vi "Database.Changeover.vi"(7 "Idx":i32, 8 "error in":errorcluster, 10 "Ref":string, 11 "Data in":T1) -> (0 "error out":errorcluster, 3 "Data out":T1)   [LabVIEW 2016]
doc: "Connect to database\n\nWabco 2017 All right reserved\nAuthor: maciej.szupienko@wabco-auto.com"
uses:
  Database.Data.ctl
  Database.Data.Status.ctl
  Database.Data.Sets.ctl
  Cache/Cache.TestSteps.Fglb.Action.ctl
  Cache/Cache.TestSteps.Fglb.TestData.ctl
  ProdaNG/Controls/ProdaNG.Process.ctl
  ProdaNG/Controls/ProdaNG.ProcessStep.ctl
  ProdaNG/Controls/ProdaNG.ProcessStepParam.ctl
  ProdaNG/Controls/ProdaNG.TestStep.ctl
  ProdaNG/Controls/ProdaNG.TestValue.ctl
  ProdaNG/Controls/ProdaNG.TestStepParam.ctl
  ProdaNG/Controls/ProdaNG.Unit.ctl
  Cache/Cache.TestSteps.Fglb.ResultData.ctl
  ProdaNG/Controls/ProdaNG.ProcessResult.ctl
  ProdaNG/Controls/ProdaNG.ProcessStepResult.ctl
  ProdaNG/Controls/ProdaNG.TestStepResult.ctl
  ProdaNG/Controls/ProdaNG.TestValueResult.ctl
  Tools/Translator/Translator.Message.ctl
  Tools/EventLog/EventLog.EventSource.ctl
  Tools/EventLog/EventLog.New(single).vi
  Global/ApplicationGlobal.vi
  Tools/EventLog/EventLog.Buffer.vi
  Tools/EventLog/EventLog.File.ReadWrite.vi
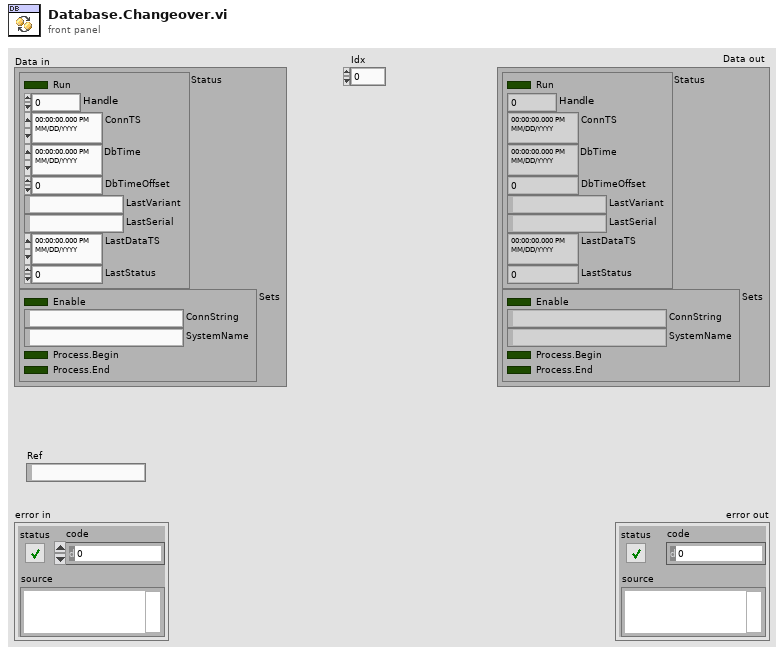
[diagram p1: front panel]
types:
  T1 = typedef "Database.Data.ctl" = cluster{"Status":T2, "Sets":T3}
  T2 = typedef "Database.Data.Status.ctl" = cluster{"Run":bool, "Handle":i32, "ConnTS":timestamp, "DbTime":timestamp, "DbTimeOffset":dbl, "LastVariant":string, "LastSerial":string, "LastDataTS":timestamp, "LastStatus":i32}
  T3 = typedef "Database.Data.Sets.ctl" = cluster{"Enable":bool, "ConnString":string, "SystemName":string, "Process.Begin":bool, "Process.End":bool}
  T4 = typedef "EventLog.EventSource.ctl" = enum16{"All", "Gui", "Cache", "PLC1", "PLC2", "PLC3", "DB", "DB01", "DB02", "DB03", "DB04", "DB05", "DB06", "DB07", "DB08", "DB09", "DB10", "DB11", "DB12", "DB13", "DB14", "DB15", "DB16"}
  T5 = typedef "Translator.Message.ctl" = enum16{"-", "Event confirmed", "Log out", "Log in", "Shutdown", "Cancel", "Start", "Continue", "Stop", "On", "Off", "OK", "NOK", "NOK %s", "This", "Prev", "Home", "Work", "In progress...", "Missing", "Empty", "Hardware failure", "Initial", "Error %d >> %s", "Error %d >> %s >> %s", "Starting %s", "Quitting %s", "Configured", "Initializing", "Quitting", "Loading", "Running %s", "Stopped", "Summary", "Do you want to continue?", "Do you want to exit?", "Log out?", "System", "All", "IDLE", "Translating...%s", "Not found", "Alarm %s", "Run", "Skip", "Abort", "Repeat", "Please wait...", "Database disconnected", "Login to database successful", "Login to database failed: %d; %s", "Get process step data for %s", "Changeover off", "Changeover into %s", "Product %s | %s found in cache with status %d at previous station", "Product %s | %s found in database with status %d at previous station", "Product %s | %s not found in cache at previous station", "Product %s | %s not found in database at previous station", "Product %s | %s found in cache with status %d at this station (%d repetion)", "Product %s | %s found in database with status %d at this station (%d repetition)", "Product %s | %s not found in cache at this station", "Product %s | %s not found in database at this station", "Product %s | %s found in cache for component %s | %s", "Product %s | %s found in database for component %s | %s", "Product not found in cache for component %s | %s", "Product not found in database for component %s | %s", "Product %s | %s connected with component %s | %s (cache)", "Product %s | %s connected with component %s | %s (database)", "New data for %s | %s (cache)", "New data for %s | %s (database)", "File %s moved (cache)", "File %s deleted (cache)", "Msg %d >> %s", "PLC LifeBit Failure", "Reconnecting DB", "Reconnecting PLC", "Free disk space is below 1GB - contact technician"}
  T6 = typedef "Cache.TestSteps.Fglb.ResultData.ctl" = cluster{"File":path, "Ref":string, "Serial":string, "Pr":T7, "PSr":T8, "TSr":cluster{"TSr":T9, "TVr":T10[]}[]}
  T7 = typedef "ProdaNG.ProcessResult.ctl" = cluster{"c_id":string, "productId":string, "processId":i32, "statusId":i32, "startTime":string, "endTime":string}
  T8 = typedef "ProdaNG.ProcessStepResult.ctl" = cluster{"c_id":string, "processResultId":string, "processStepId":i32, "statusId":i32, "operatorId":i32, "startTime":string, "endTime":string}
  T9 = typedef "ProdaNG.TestStepResult.ctl" = cluster{"c_id":string, "processStepResultId":string, "testStepId":i32, "statusId":i32}
  T10 = typedef "ProdaNG.TestValueResult.ctl" = cluster{"c_id":string, "testStepResultId":string, "testValueId":i32, "result":dbl, "statusId":i32, "contentId":string}
  T11 = typedef "Cache.TestSteps.Fglb.TestData.ctl" = cluster{"Ref":string, "Desc":string, "P":T12, "PS":T13, "PP":T14[], "TS":cluster{"TS":T15, "TV":T16[], "TP":T17[]}[], "Units":T18[]}
  T12 = typedef "ProdaNG.Process.ctl" = cluster{"i_id":i32, "productionLineId":i32, "releaseId":i32, "contentId":string, "previewId":string, "mdReason":string, "mdUser":string, "mdTime":string, "description":string}
  T13 = typedef "ProdaNG.ProcessStep.ctl" = cluster{"i_id":i32, "processId":i32, "systemId":i32, "releaseId":i32, "processSequence":i32, "limitYellow":dbl, "limitRed":dbl, "mdReason":string, "mdUser":string, "mdTime":string, "filename":string, "transfer":string, "description":string}
  T14 = typedef "ProdaNG.ProcessStepParam.ctl" = cluster{"i_id":i32, "processStepId":i32, "unitId":i32, "contentId":string, "previewId":string, "value":dbl, "valueText":string, "paramSequence":i32, "history":i32, "mdReason":string, "mdUser":string, "mdTime":string, "description":string}
  T15 = typedef "ProdaNG.TestStep.ctl" = cluster{"i_id":i32, "processStepId":i32, "testSequence":i32, "testOrder":i32, "mdReason":string, "mdUser":string, "mdTime":string, "description":string}
  T16 = typedef "ProdaNG.TestValue.ctl" = cluster{"i_id":i32, "testStepId":i32, "releaseId":i32, "unitId":i32, "contentId":string, "previewId":string, "maximum":dbl, "minimum":dbl, "valueText":string, "testValueSequence":i32, "history":i32, "mdReason":string, "mdUser":string, "mdTime":string, "description":string}
  T17 = typedef "ProdaNG.TestStepParam.ctl" = cluster{"i_id":i32, "testStepId":i32, "unitId":i32, "contentId":string, "previewId":string, "value":dbl, "valueText":string, "paramSequence":i32, "history":i32, "mdReason":string, "mdUser":string, "mdTime":string, "description":string}
  T18 = typedef "ProdaNG.Unit.ctl" = cluster{"i_id":i32, "name":string, "mdReason":string, "mdUser":string, "mdTime":string, "description":string}
  T19 = typedef "Cache.TestSteps.Fglb.Action.ctl" = enum16{"init", "add", "get"}
  T20 = typedef "Database.Data.Variant.Sets.ctl" = cluster{"PrevStations":string[], "ThisStations":string[]}
  T21 = typedef "ProdaNG.Identification.ctl" = cluster{"processId":i32, "systemId":i32, "processStepId":i32, "wabcoPartId":i32}
  T22 = cluster{"TestStep":T15, "TestStepValues":T16[], "TestStepParams":T17[]}
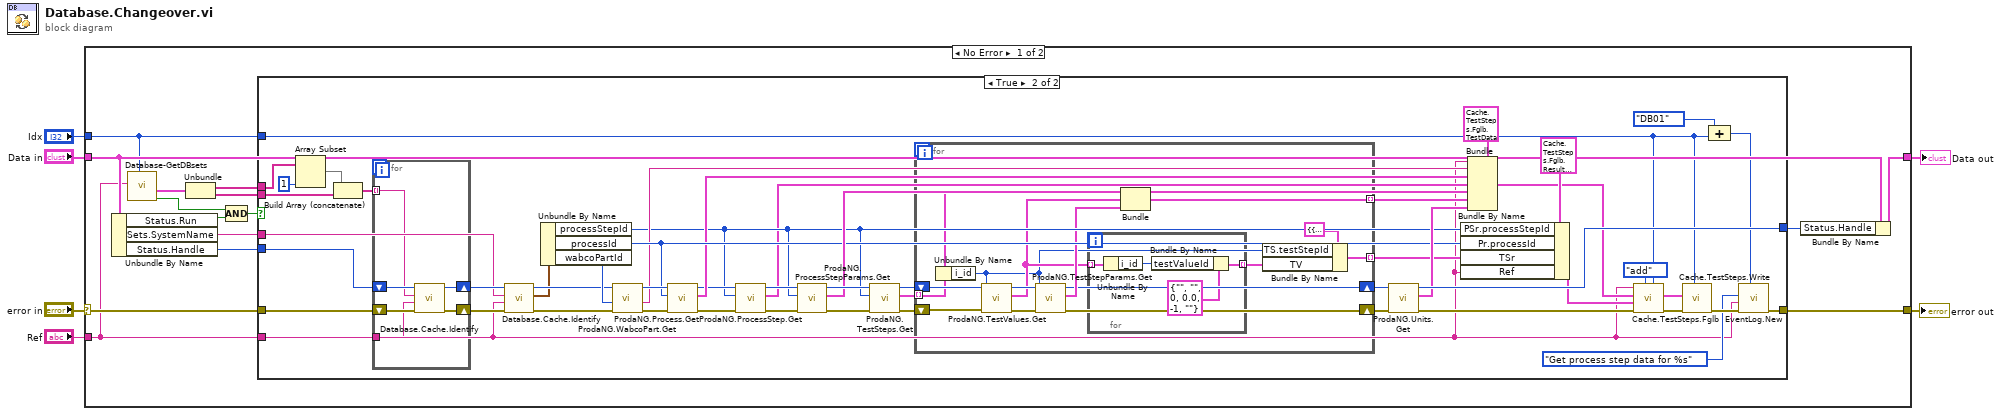
[diagram p0: block diagram]
diagram:
  n1 = case shown="No Error" "error in" {
    selector: "error in" -> [w21 w101]
    tunnel: [w7 w101] -> w6
    tunnel: "Data in" -> [w18 w100]
    tunnel: "Idx" -> [w8 _]
    tunnel: [w16 w100] -> w2
    tunnel: "Ref" -> [w12 _]
    frame No Error {
      n2 = Unbundle By Name(w18) -> ("Status.Run"=w11:bool, "Sets.SystemName"=w20:string, "Status.Handle"=w19:i32)
      n3 = call "Database-GetDBsets.vi"("Idx"=w8, "Variant"=w12) -> ("Found"=w10:bool, "Variant Sets"=w15:T20)  [unwired: 5 in, 3 out]
      n4 = Unbundle(w15) -> ("PrevStations"=w14:string[], "ThisStations"=w13:string[])
      n5 = Compound Arithmetic op=AND(w10, w11) -> (w9:bool)
      n6 = case shown="True" w9 {
        tunnel: w21 -> [w22 w43]
        tunnel: [w22 w29] -> w7
        tunnel: w14 -> [_ w33]
        tunnel: w20 -> [_ w34]
        tunnel: w19 -> [w23 w40]
        tunnel: [w23 w75] -> w17
        tunnel: w13 -> [_ w42]
        tunnel: w12 -> [_ w24]
        tunnel: w8 -> [_ w27]
        frame False {
        }
        frame True {
          n7 = Array Subset(array=w33, length=1) -> (w32:string[])  [unwired: 1 in]
          n8 = Build Array (concatenate)(w32, w42) -> (w41:string[])
          n9 = for {
            tunnel: w41 -> [w76] mode=indexing
            shift-right: [w80] -> w38
            shift-left: w40 -> [w79]
            tunnel: w24 -> [w77]
            shift-right: [w81] -> w39
            shift-left: w43 -> [w78]
            n10 = call "Database.Cache.Identify.vi"("error in (no error)"=w78, "Variant"=w77, "SystemName"=w76, "DB Handle in"=w79) -> ("error out"=w81:errorcluster, "DB Handle out"=w80:i32)  [unwired: 5 in, 1 out]
          }
          n11 = call "Database.Cache.Identify.vi"("error in (no error)"=w39, "Variant"=w24, "SystemName"=w34, "DB Handle in"=w38) -> ("error out"=w37:errorcluster, "SytemID"=w35:T21, "DB Handle out"=w36:i32)  [unwired: 5 in]
          n12 = Unbundle By Name(w35) -> ("processStepId"=w45:i32, "processId"=w55:i32, "wabcoPartId"=w74:i32)
          n13 = call "ProdaNG.WabcoPart.Get.vi"("error in (no error)"=w37, "WabcoPartId (-1: use WabcoNumber)"=w74, "dbHandleIn"=w36) -> ("error out"=w72:errorcluster, "ProductName"=w52:string, "dbHandle"=w73:i32)  [unwired: 5 in, 1 out]
          n14 = call "ProdaNG.Process.Get.vi"("error in (no error)"=w72, "processId"=w55, "dbHandleIn"=w73) -> ("error out"=w48:errorcluster, "Process"=w53:T12, "dbHandle"=w49:i32)  [unwired: 5 in, 1 out]
          n15 = call "ProdaNG.ProcessStep.Get.vi"("error in (no error)"=w48, "processStepId"=w45, "dbHandleIn"=w49) -> ("error out"=w47:errorcluster, "ProcessStep"=w44:T13, "dbHandle"=w46:i32)  [unwired: 6 in]
          n16 = call "ProdaNG.ProcessStepParams.Get.vi"("error in (no error)"=w47, "processStepId"=w45, "dbHandleIn"=w46) -> ("error out"=w70:errorcluster, "ProcStepParams"=w60:T14[], "dbHandle"=w69:i32)  [unwired: 6 in]
          n17 = call "ProdaNG.TestSteps.Get.vi"("error in (no error)"=w70, "processStepId"=w45, "dbHandleIn"=w69) -> ("error out"=w68:errorcluster, "TestSteps"=w66:T15[], "dbHandle"=w67:i32)  [unwired: 6 in]
          n18 = for {
            shift-right: [w91] -> w64
            shift-left: w68 -> [w95]
            tunnel: w66 -> [w83] mode=indexing
            tunnel: [w90] -> w65 mode=indexing
            tunnel: [w84] -> w56 mode=indexing
            shift-right: [w82] -> w63
            shift-left: w67 -> [w94]
            n19 = Unbundle By Name(w83) -> ("i_id"=w86:i32)
            n20 = call "ProdaNG.TestValues.Get.vi"("error in (no error)"=w95, "testStepId"=w86, "dbHandleIn"=w94) -> ("error out"=w92:errorcluster, "TestStepValues"=w87:T16[], "dbHandle"=w93:i32)  [unwired: 6 in]
            n21 = call "ProdaNG.TestStepParams.Get.vi"("error in (no error)"=w92, "testStepId"=w86, "dbHandleIn"=w93) -> ("error out"=w91:errorcluster, "TestStepParams"=w89:T17[], "dbHandle"=w82:i32)  [unwired: 6 in]
            n22 = for {
              tunnel: w87 -> [w99] mode=indexing
              tunnel: [w96] -> w88 mode=indexing
              n23 = Unbundle By Name(w99) -> ("i_id"=w98:i32)
              n24 = Bundle By Name(cluster=T10 {"c_id"="", "testStepResultId"="", "testValueId"=0, "result"=0.0, "statusId"=-1, "contentId"=""} ("TV"), "testValueId"=w98) -> (w96:T10)
            }
            n25 = Bundle("TestStep"=w83, "TestStepValues"=w87, "TestStepParams"=w89) -> (w90:T22)  [unwired: 1 in]
            n26 = Bundle By Name(cluster=cluster{"TS":T9, "TV":T10[]} {"TS"={"c_id"="", "processStepResultId"="", "testStepId"=0, "statusId"=-1}, "TV"=[]} ("Cluster"), "TS.testStepId"=w86, "TV"=w88) -> (w84:cluster{"TS":T9, "TV":T10[]})
          }
          n27 = call "ProdaNG.Units.Get.vi"("error in (no error)"=w64, "dbHandleIn"=w63) -> ("error out"=w57:errorcluster, "units"=w62:T18[], "dbHandle"=w75:i32)  [unwired: 6 in, 1 out]
          n28 = Bundle By Name(cluster=T6 {"File"=path "", "Ref"="", "Serial"="", "Pr"={"c_id"="", "productId"="", "processId"=0, "statusId"=0, "startTime"="", "endTime"=""}, "PSr"={"c_id"="", "processResultId"="", "processStepId"=0, "statusId"=0, "operatorId"=0, "startTime"="", "endTime"=""}, "TSr"=[]} ("Result in"), "PSr.processStepId"=w45, "Pr.processId"=w55, "TSr"=w56, "Ref"=w24) -> (w58:T6)
          n29 = Bundle(cluster=T11 {"Ref"="", "Desc"="", "P"={"i_id"=0, "productionLineId"=0, "releaseId"=0, "contentId"="", "previewId"="", "mdReason"="", "mdUser"="", "mdTime"="", "description"=""}, "PS"={"i_id"=0, "processId"=0, "systemId"=0, "releaseId"=0, "processSequence"=0, "limitYellow"=0.0, "limitRed"=0.0, "mdReason"="", "mdUser"="", "mdTime"="", "filename"="", "transfer"="", "description"=""}, "PP"=[], "TS"=[], "Units"=[]} ("TestStep in"), "Ref"=w24, "Desc"=w52, "P"=w53, "PS"=w44, "PP"=w60, "TS"=w65, "Units"=w62) -> (w54:T11)
          n30 = call "Cache.TestSteps.Fglb.vi"("SystemIdx"=w27, "Action (get)"=Cache.TestSteps.Fglb.Action."add", "error in (no error)"=w57, "Result in"=w58, "Test in"=w54, "Variant"=w24) -> ("error out"=w51:errorcluster, "Test out"=w50:T11)  [unwired: 2 in, 2 out]
          n31 = call "Cache.TestSteps.Write.vi"("Idx"=w27, "error in (no error)"=w51, "TS in"=w50) -> ("error out"=w30:errorcluster)  [unwired: 8 in]
          n32 = Compound Arithmetic op=ADD(EventLog.EventSource."DB01" ("Source (All)"), w27) -> (w25:i32)
          n33 = call-poly "EventLog.New.vi"("Source (All)"=w25, "error in (no error)"=w30, "Arg"=w24, "Message (-)"=Translator.Message."Get process step data for %s") -> ("error out"=w29:errorcluster)  [unwired: 6 in, 1 out]
        }
      }
      n34 = Bundle By Name(cluster=w18, "Status.Handle"=w17) -> (w16:T1)
    }
    frame Error {
    }
  }
  "error out" <- w6
  "Data out" <- w2
